vi "RegDataChannel.vi"(8 "error in":T1, 10 "buffersize":i32, 11 "channel":T2=1 items=["Channel 0", "Channel 1", "Channel 2", "Channel 3", "Channel 4", "Channel 5", "Channel 6", "Channel 7", "Channel 8", "Channel 9", "Channel 10", "Channel 11", "Channel 12", "Channel 13"]) -> (0 "error out":T1)   [LabVIEW 2016]
doc: "Registers a data channel, which enables the reception of data over the specified 'channel'. The buffer size must be at least one frame size (see getFrameSize.vi) and greater than 129."
uses:
  Controls/Channel_Selection.ctl
  Controls/Error_Out.ctl
  Files_ASC500/DLL/ASC500_RemoteControlV27.dll
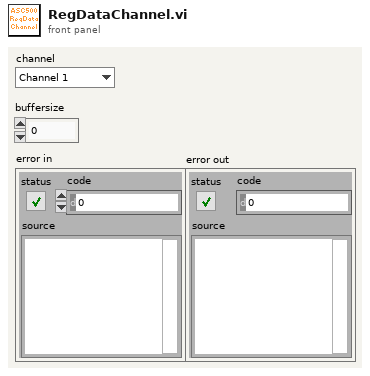
[diagram p1: front panel]
types:
  T1 = typedef "Error_Out.ctl" = errorcluster
  T2 = typedef "Channel_Selection.ctl" = i32
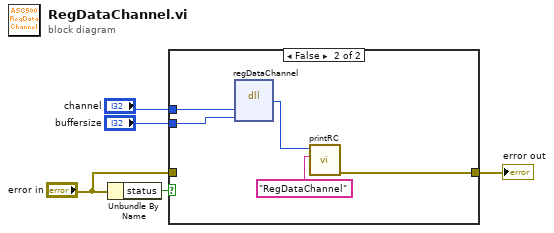
[diagram p0: block diagram]
diagram:
  n1 = Unbundle By Name("error in") -> ("status"=w5:bool)
  n2 = case shown="False" w5 {
    tunnel: [w6 w9] -> w4
    tunnel: "channel" -> [_ w11]
    tunnel: "error in" -> [w6 _]
    tunnel: "buffersize" -> [_ w7]
    frame True {
    }
    frame False {
      n3 = dll-call lib="G:/SCMOperations/Share/ELE/Produkt Information/ASC500/04 Remote Control/02 development versions/2018Nov06/Files_ASC500/DLL/ASC500_RemoteControlV27.dll" fn="regDataChannel"("Channel"=w11, "buffersize"=w7) -> ("return type"=w10:i32)  [unwired: 5 in, 2 out]
      n4 = call "printRC.vi"("additional information"="RegDataChannel", "RC"=w10) -> ("error out"=w9:T1)  [unwired: 9 in]
    }
  }
  "error out" <- w4
